vi "小时数据发送 (子VI).vi"(11 "数值":i32) -> (0 "error out":errorcluster, 3 "超时退出":bool)   [LabVIEW 2016, in "数据传输系统-05.lvlib"]
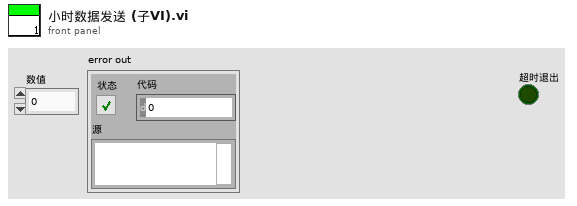
[diagram p1: front panel]
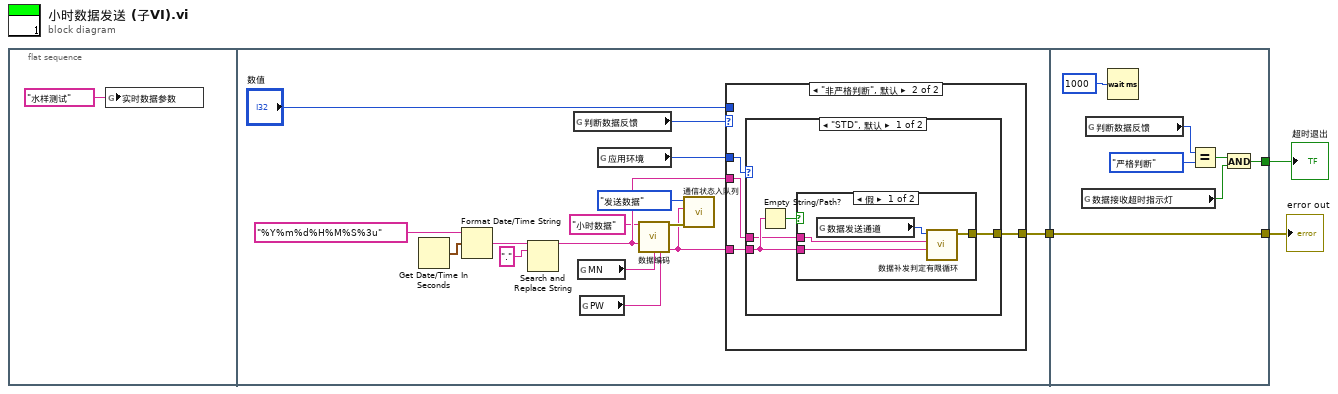
[diagram p0: block diagram]
diagram:
  n1 = flat-sequence {
    tunnel: [w8] -> w2
    tunnel: [w38] -> w3
    tunnel: w2 -> [w38]
    tunnel: [w32] -> w1
    frame #0 {
      n2 = global write "全局 实时数据参数.vi" "实时数据参数"("水样测试" ("实时数据参数")) -> ()
    }
    frame #1 {
      n3 = Get Date/Time In Seconds() -> (seconds since 1Jan1904=w12:timestamp)
      n4 = Format Date/Time String(time format string (%c)="%Y%m%d%H%M%S%3u" ("时间格式字符串(%c)"), seconds (now)=w12) -> (date/time string=w11:string)  [unwired: 1 in]
      n5 = Search and Replace String(input string=w11, search string="." ("搜索字符串")) -> (result string=w19:string)  [unwired: 6 in, 3 out]
      n6 = global read "断电保存全局.vi" "判断数据反馈"() -> (w18:enum16{"非严格判断", "严格判断", "不判断"})
      n7 = global read "断电保存全局.vi" "MN"() -> (w15:string)
      n8 = global read "断电保存全局.vi" "PW"() -> (w16:string)
      n9 = global read "断电保存全局.vi" "应用环境"() -> (w7:enum16{"STD", "GB212"})
      n10 = call "数据编码.vi"("table输入"="小时数据" ("新元素/子数组"), "QN"=w19, "MN"=w15, "PW"=w16) -> ("错误常量"=w17:errorcluster, "通讯包字符串"=w5:string)  [unwired: 10 in]
      n11 = call "通信状态入队列.vi"("错误输入（无错误）"=w17, "发送报文"=w5, "枚举"=enum16{"打开连接", "发送数据", "读取数据", "数据处理", "关闭连接"}."发送数据") -> ()  [unwired: 8 in, 1 out]
      n12 = case shown="\"非严格判断\", 默认" w18 {
        tunnel: [_ w23] -> w8
        tunnel: w5 -> [_ w22]
        tunnel: "数值" -> [_ _]
        tunnel: w19 -> [_ w21]
        tunnel: w7 -> [_ w20]
        frame "不判断" {
        }
        frame "非严格判断", Default {
          n13 = case shown="\"STD\", 默认" w20 {
            tunnel: [w26 _] -> w23
            tunnel: w22 -> [w25 _]
            tunnel: w21 -> [w24 _]
            frame "STD", Default {
              n14 = Empty String/Path?(string/path=w25) -> (empty?=w27:bool)
              n15 = case shown="假" w27 {
                tunnel: [w31 _] -> w26
                tunnel: w25 -> [w30 _]
                tunnel: w24 -> [w28 _]
                frame False {
                  n16 = global read "断电保存全局.vi" "数据发送通道"() -> (w29:enum16{"TCP", "VISA"})
                  n17 = call "数据补发判定有限循环.vi"("数据输入"=w30, "QN"=w28, "数据发送通道"=w29) -> ("error out"=w31:errorcluster)  [unwired: 8 in]
                }
                frame True {
                }
              }
            }
            frame "GB212" {
            }
          }
        }
      }
    }
    frame #2 {
      n18 = global read "全局 数据发送重叠.vi" "数据接收超时指示灯"() -> (w33:bool)
      n19 = global read "断电保存全局.vi" "判断数据反馈"() -> (w36:enum16{"非严格判断", "严格判断", "不判断"})
      n20 = Wait (ms)(milliseconds to wait=u32 1000 ("等待时间（毫秒）")) -> ()  [unwired: 1 out]
      n21 = Equal?(x=w36, y=enum16{"非严格判断", "严格判断", "不判断"}."严格判断") -> (x = y?=w34:bool)
      n22 = And(x=w34, y=w33) -> (x .and. y?=w32:bool)
    }
  }
  "error out" <- w3
  "超时退出" <- w1
